vi "探测器列表-累积校准.vi"(6 "元素名[]-探测器信息":string[](array[string]), 7 "元素名[]-累积记录":string[](array[string]), 8 "error in (no error)":errorcluster, 9 "表名-设备表":string, 10 "名称":string, 11 "数据库引用":T1) -> (0 "error out":errorcluster, 2 "校准值":dbl, 3 "connection reference out":T1)   [LabVIEW 2017]
uses:
  <vilib>/addons/database/Connection.llb/Conn ObjectReference.ctl
  <vilib>/addons/database/NI_Database_API.lvlib
panel:
  out "Result 2":string caption="update sql结果"
  out "Result":string caption="sum() sql结果"
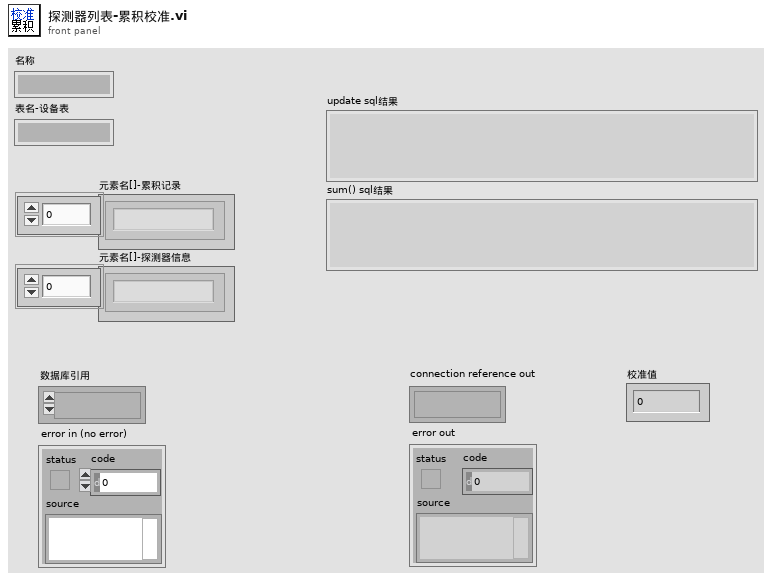
[diagram p1: front panel]
types:
  T1 = typedef "NI_Database_API.lvlib/Conn ObjectReference.ctl" = refnum<k1>
  T2 = typedef "单条累积记录.ctl" = cluster{"起始时间":timestamp, "结束时间":timestamp, "累积剂量":dbl}
  T3 = typedef "探测器信息.ctl" = cluster{"网络地址":string, "名称":string, "备注":string, "累积剂量":dbl, "累积限值":dbl, "硬件剂量率限值":T4, "剂量率限值1":dbl, "剂量率限值2":dbl, "报警方式":T5}
  T4 = typedef "探头剂量率限值选择.ctl" = enum16{"一级限值", "二级限值"}
  T5 = typedef "报警方式选择.ctl" = enum16{"常报警", "自动静音", "手动静音"}
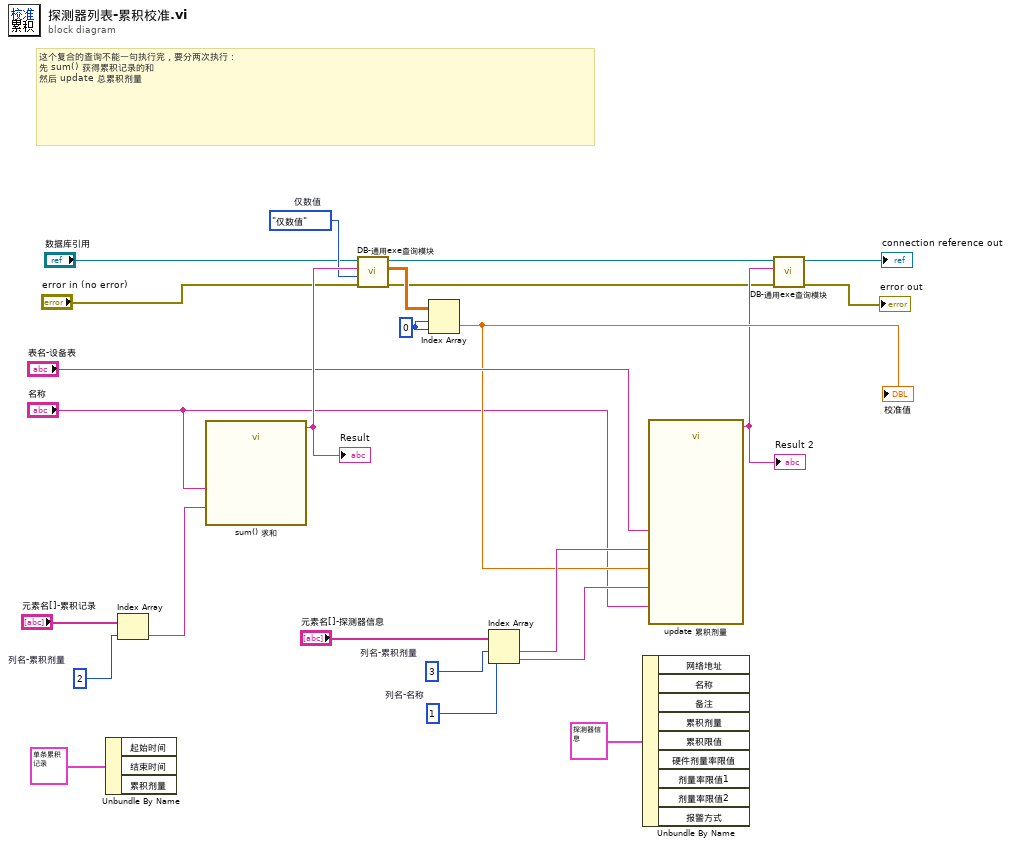
[diagram p0: block diagram]
diagram:
  w10 = 1  # 列名-名称
  w13 = 3  # 列名-累积剂量
  w15 = 0 ("索引 (行)")
  w17 = enum16{"仅数值", "仅字符串", "数值与字符串", "不转换", "不抓取"}."仅数值"  # 仅数值
  w20 = 2  # 列名-累积剂量
  # "这个复合的查询不能一句执行完，要分两次执行：\n先 sum() 获得累积记录的和\n然后 update 总累积剂量"
  n1 = Unbundle By Name(T2 {"起始时间"=timestamp(0 s since 1904-01-01), "结束时间"=timestamp(0 s since 1904-01-01), "累积剂量"=0.0} ("累积记录")) -> ()  [unwired: 3 out]
  n2 = Index Array(array="元素名[]-累积记录", index=w20) -> (element=w19:string)
  n3 = call "sum() 求和"("列名-累积记录值"=w19, "表名-设备名称"="名称") -> ("Result"=w18:string)  [unwired: 12 in, 1 out]
  "Result" <- w18
  n4 = call "DB-通用exe查询模块.vi"("error in (no error)"="error in (no error)", "解析模式"=w17, "SQL query"=w18, "数据库连接引用"="数据库引用") -> ("error out"=w4:errorcluster, "数值数据"=w16:dbl[][], "数据库连接引用out"=w5:T1)  [unwired: 3 in, 2 out]
  n5 = Index Array(array=w16, index (row)=w15, index (col)=w15) -> (element=w11:dbl)
  "校准值" <- w11
  n6 = Index Array(array="元素名[]-探测器信息", index #1=w13, index #2=w10) -> (element #1=w12:string, element #2=w9:string)
  n7 = Unbundle By Name(T3 {"网络地址"="", "名称"="", "备注"="", "累积剂量"=0.0, "累积限值"=0.0, "硬件剂量率限值"=enum."一级限值", "剂量率限值1"=0.0, "剂量率限值2"=0.0, "报警方式"=enum."常报警"} ("探测器信息")) -> ()  [unwired: 9 out]
  n8 = call "update 累积剂量"("列名-名称"=w9, "表名-设备表"="表名-设备表", "列名-累积剂量"=w12, "校准值"=w11, "名称"="名称") -> ("Result"=w7:string)  [unwired: 9 in, 1 out]
  "Result 2" <- w7
  n9 = call "DB-通用exe查询模块.vi"("error in (no error)"=w4, "SQL query"=w7, "数据库连接引用"=w5) -> ("error out"=→"error out":errorcluster, "数据库连接引用out"=→"connection reference out":T1)  [unwired: 4 in, 3 out]
